vi "1002_FireAt1015EveryDay.vi"(8 "error in (no error)":errorcluster) -> (0 "error out":errorcluster)   [LabVIEW 2013]
uses:
  <vilib>/addons/_JKI Toolkits/Caraya/classes/Assert/Assert True.vi
  source/Cron/Create Cron Expression.vi
  source/Cron/Compute Next Cron.vi
  source/Cron.Unix/Cron.Unix.lvclass
  <vilib>/addons/_JKI Toolkits/Caraya/classes/Test/Test.lvclass
  <vilib>/addons/_JKI Toolkits/Caraya/classes/Assert/Assert.lvclass
  source/openCron.lvlib
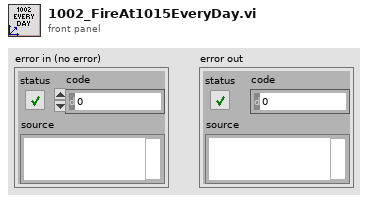
[diagram p1: front panel]
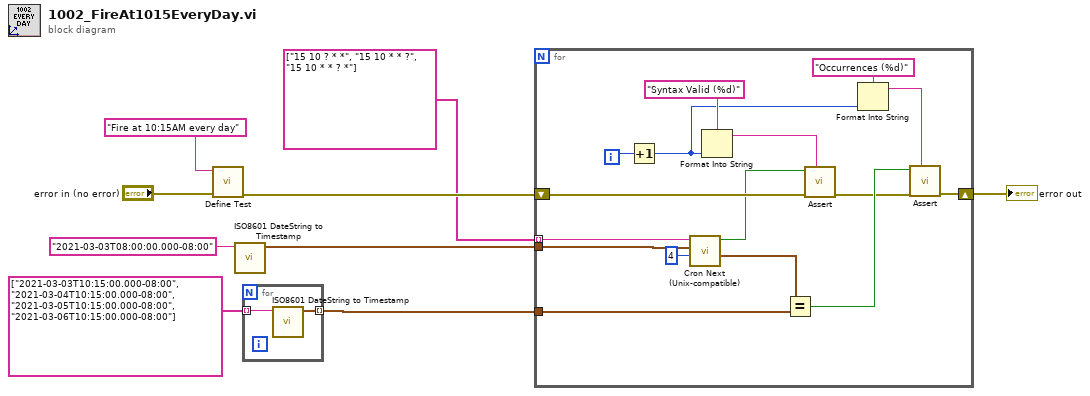
[diagram p0: block diagram]
diagram:
  n1 = call <vilib>:"Define Test.vi"("error in (no error)"="error in (no error)", "Label (VI Title)"="Fire at 10:15AM every day") -> ("error out"=w7:errorcluster)  [unwired: 8 in, 1 out]
  n2 = call <vilib>:"ISO8601 DateString to Timestamp.vi"("ISO8601 Date String"="2021-03-03T08:00:00.000-08:00" ("Expression")) -> ("Timestamp"=w2:timestamp)  [unwired: 8 in, 2 out]
  n3 = for {
    tunnel: string[] ["2021-03-03T10:15:00.000-08:00", "2021-03-04T10:15:00.000-08:00", "2021-03-05T10:15:00.000-08:00", "2021-03-06T10:15:00.000-08:00"] -> [w11] mode=indexing
    tunnel: [w10] -> w1 mode=indexing
    n4 = call <vilib>:"ISO8601 DateString to Timestamp.vi"("ISO8601 Date String"=w11) -> ("Timestamp"=w10:timestamp)  [unwired: 8 in, 2 out]
  }
  n5 = for {
    tunnel: w1 -> [w24]
    tunnel: string[] ["15 10 ? * *", "15 10 * * ?", "15 10 * * ? *"] -> [w16] mode=indexing
    shift-right: [w27] -> w9
    shift-left: w7 -> [w23]
    tunnel: w2 -> [w12]
    i -> [w22]
    n6 = Increment(x=w22) -> (x+1=w18:i32)
    n7 = call "Cron Next (Unix-compatible).vi"("Nb Occurences (min: 1)"=u16 4, "Reference timestamp (Now)"=w12, "Cron Expression"=w16) -> ("Occurences"=w14:timestamp[], "syntax valid?"=w13:bool)  [unwired: 6 in, 1 out]
    n8 = Format Into String(format string="Syntax Valid (%d)" ("Label (VI Title)"), w18) -> (resulting string=w20:string)  [unwired: 2 in, 1 out]
    n9 = Equal?(x=w14, y=w24) -> (x = y?=w26:bool)
    n10 = call-poly <vilib>:"Assert.vi"("Label"=w20, "error in (no error)"=w23, "True?"=w13) -> ("error out"=w25:errorcluster)  [unwired: 7 in, 1 out]
    n11 = Format Into String(format string="Occurrences (%d)" ("Label (VI Title)"), w18) -> (resulting string=w17:string)  [unwired: 2 in, 1 out]
    n12 = call-poly <vilib>:"Assert.vi"("Label"=w17, "error in (no error)"=w25, "True?"=w26) -> ("error out"=w27:errorcluster)  [unwired: 7 in, 1 out]
  }
  "error out" <- w9
